vi "Determine Scan Name.vi"(8 "error in (no error)":errorcluster, 11 "Model in":refnum<class "Model.lvclass">) -> (0 "error out":errorcluster, 2 "Scan Name":string, 3 "Model out":refnum<class "Model.lvclass">)   [LabVIEW 2015, in "Model.lvclass"]
uses:
  Model.lvclass
  Model.lvclass/Model.ctl
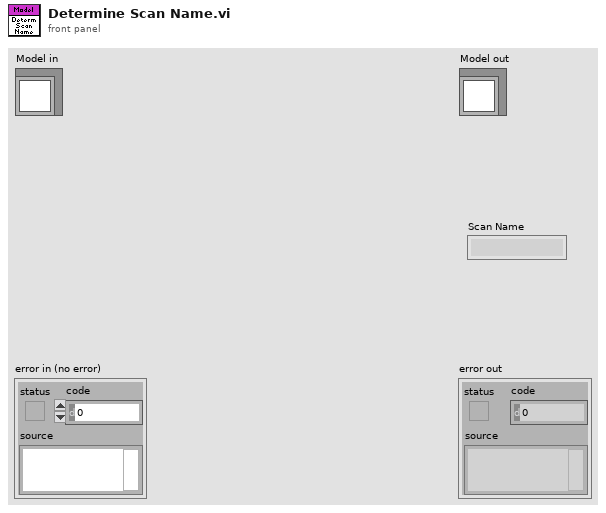
[diagram p1: front panel]
types:
  T1 = typedef "FAMT Typedefs.lvlib/Actuator Types.ctl" = enum16{"Single", "Dual"}
  T2 = typedef "FAMT Typedefs.lvlib/Waveform Settings.ctl" = cluster{"Sample Count":u32, "Amplitude":dbl, "Offset":dbl, "Frequency":dbl[unit], "Waveform":T3, "F1":dbl[unit], "F2":dbl[unit], "Duty Cycle":dbl, "ILC Rate":dbl[unit], "Ramp Time":dbl[unit], "Hold Time":dbl[unit], "Settling Time":dbl[unit], "Delay":dbl[unit]}
  T3 = typedef "FAMT Typedefs.lvlib/Waveform Types.ctl" = enum16{"Sine", "Triangle", "Square", "Sawtooth", "Chirp", "Gaussian", "Trapezoid"}
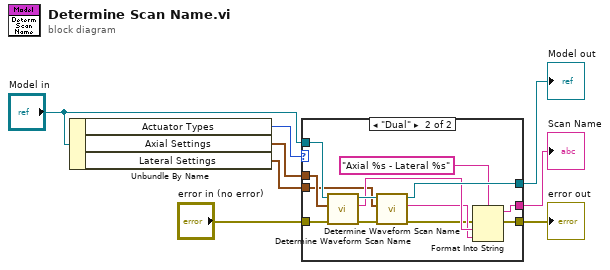
[diagram p0: block diagram]
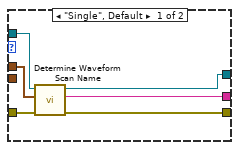
[diagram p2: hidden frame]
diagram:
  n1 = Unbundle By Name("Model in") -> ("Actuator Types"=w8:T1, "Axial Settings"=w3:T2, "Lateral Settings"=w1:T2)
  n2 = case shown="\"Dual\"" w8 {
    tunnel: "Model in" -> [w14 w27]
    tunnel: [w13 w25] -> w6
    tunnel: [w12 w19] -> w5
    tunnel: "error in (no error)" -> [w11 w17]
    tunnel: w3 -> [w10 w16]
    tunnel: [w9 w23] -> w2
    tunnel: w1 -> [_ w15]
    frame "Single", Default {
      n3 = call "Determine Waveform Scan Name.vi"("error in (no error)"=w11, "Waveform Settings"=w10, "Model in"=w14) -> ("error out"=w12:errorcluster, "Waveform Scan Name"=w9:string, "Model out"=w13:refnum<class "Model.lvclass">)  [unwired: 6 in]
    }
    frame "Dual" {
      n4 = call "Determine Waveform Scan Name.vi"("error in (no error)"=w17, "Waveform Settings"=w16, "Model in"=w27) -> ("error out"=w18:errorcluster, "Waveform Scan Name"=w22:string, "Model out"=w26:refnum<class "Model.lvclass">)  [unwired: 6 in]
      n5 = call "Determine Waveform Scan Name.vi"("error in (no error)"=w18, "Waveform Settings"=w15, "Model in"=w26) -> ("error out"=w20:errorcluster, "Waveform Scan Name"=w21:string, "Model out"=w25:refnum<class "Model.lvclass">)  [unwired: 6 in]
      n6 = Format Into String(format string="Axial %s - Lateral %s", error in=w20, w22, w21) -> (resulting string=w23:string, error out=w19:errorcluster)  [unwired: 1 in]
    }
  }
  "error out" <- w5
  "Model out" <- w6
  "Scan Name" <- w2
